vi "Reply.vi"(8 "error in (no error)":errorcluster, 10 "Response":string, 11 "MicronMessage in":refnum<class "GRPCMessage.lvclass">) -> (0 "error out":errorcluster, 3 "MicronMessage out":refnum<class "GRPCMessage.lvclass">)   [LabVIEW 2019, in "MicronGRPCServer.lvlib" / "GRPCMessage.lvclass"]
uses:
  GRPCMessage.lvclass
  Service/Generated/MicronGRPCGeneratedServer/RPC Messages/micronGrpc_MessageReply.ctl
  Service/Generated/MicronGRPCGeneratedServer/RPC Messages/micronGrpc_MessageReply_Status.ctl
  GRPCMessage.lvclass/GRPCMessage.ctl
  Service/Generated/MicronGRPCGeneratedServer/RPC Service/MicronGRPC/MicronGRPC.lvclass
  Service/Generated/MicronGRPCGeneratedServer/MicronGRPCGeneratedServer.lvlib
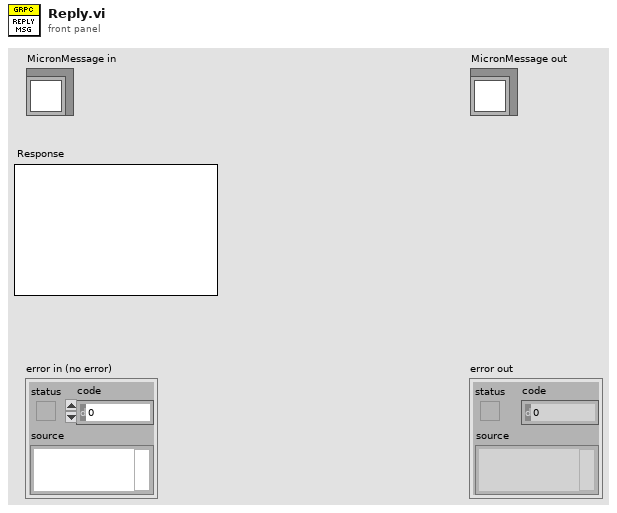
[diagram p1: front panel]
types:
  T1 = typedef "MicronGRPCGeneratedServer.lvlib/micronGrpc_MessageReply.ctl" = cluster{"payload":string, "status":T2}
  T2 = typedef "MicronGRPCGeneratedServer.lvlib/micronGrpc_MessageReply_Status.ctl" = cluster{"code":i32, "is_error":bool, "desc":string}
  T3 = typedef "grpc-lvsupport-release.lvlib/grpcId.ctl" = u64
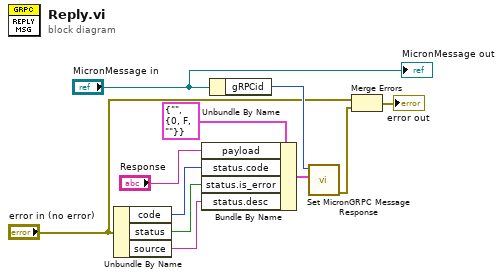
[diagram p0: block diagram]
diagram:
  n1 = Unbundle By Name("error in (no error)") -> ("code"=w9:i32, "status"=w8:bool, "source"=w7:string)
  n2 = Bundle By Name(cluster=T1 {"payload"="", "status"={"code"=0, "is_error"=FALSE, "desc"=""}} ("Message Data"), "payload"="Response", "status.code"=w9, "status.is_error"=w8, "status.desc"=w7) -> (w1:T1)
  n3 = Unbundle By Name("MicronMessage in") -> ("gRPCid"=w11:T3)
  n4 = call "Set MicronGRPC Message Response.vi"("Message Data"=w1, "gRPCid in"=w11) -> ("error out"=w5:errorcluster)  [unwired: 9 in]
  n5 = Merge Errors("error in (no error)", w5) -> (→"error out":errorcluster)
  "MicronMessage out" <- "MicronMessage in"
